vi "Ball Intake Piston.vi"   [LabVIEW 2019]
uses:
  <vilib>/Rock Robotics/WPI/Solenoid/WPI_SolenoidValue.ctl
  <vilib>/Rock Robotics/WPI/Solenoid/Deprecated/WPI_SolenoidGetBool.vi
  <vilib>/Rock Robotics/WPI/Solenoid/WPI_SolenoidSetEnum.vi
types:
  T1 = typedef "WPI_SolenoidValue.ctl" = enum16{"Off", "On", "Forward", "Reverse"}
  T2 = typedef "WPI_SolenoidDevRef.ctl" = cluster{"DevStatus":errorcluster, "Pneumatics Control Module":u8, "Forward Solenoid Channel":T3, "Reverse Solenoid Channel":T3}
  T3 = typedef "WPI_SolenoidChannel.ctl" = enum8{"Solenoid 0", "Solenoid 1", "Solenoid 2", "Solenoid 3", "Solenoid 4", "Solenoid 5", "Solenoid 6", "Solenoid 7", "Invalid"}
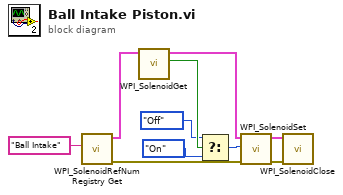
[diagram p0: block diagram]
diagram:
  n1 = call <vilib>:"WPI_SolenoidRefNum Registry Get.vi"("refnum name"="Ball Intake") -> ("error out"=w4:errorcluster, "SolenoidDevRef"=w9:T2)  [unwired: 9 in]
  n2 = call-poly <vilib>:"WPI_SolenoidGet.vi"("SolenoidDevRef"=w9) -> ("Value"=w8:bool, "SolenoidDevRef"=w10:T2)  [unwired: 8 in, 1 out]
  n3 = Select(t=WPI_SolenoidValue."Off" ("Value"), s=w8, f=WPI_SolenoidValue."On" ("Value")) -> (s? t:f=w7:T1)
  n4 = call-poly <vilib>:"WPI_SolenoidSet.vi"("error in (no error)"=w4, "Value"=w7, "SolenoidDevRef"=w10) -> ("error out"=w3:errorcluster, "SolenoidDevRef"=w2:T2)  [unwired: 7 in]
  n5 = call <vilib>:"WPI_SolenoidClose.vi"("error in (no error)"=w3, "SolenoidDevRef"=w2) -> ()  [unwired: 9 in, 1 out]
